vi "attempt path fix.vi"(9 "other possible paths":path[](array[path]), 10 "working directory":path, 11 "path to fix":path) -> (3 "path out":path)   [LabVIEW 2018]
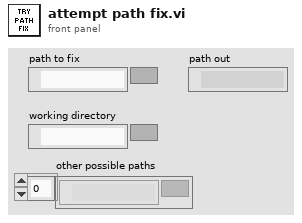
[diagram p1: front panel]
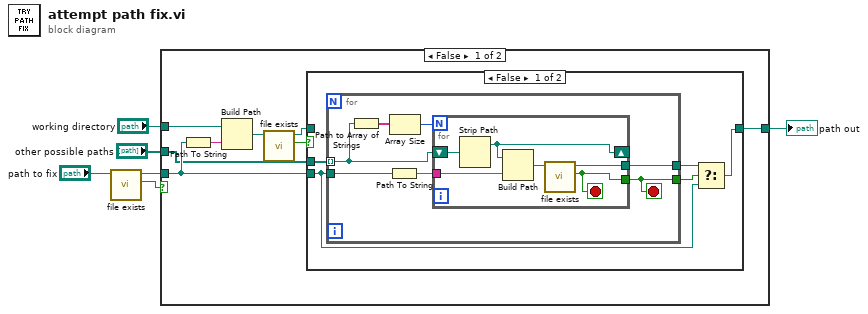
[diagram p0: block diagram]
diagram:
  n1 = call "file exists.vi"("Path in"="path to fix") -> ("file exists"=w5:bool, "Path out"=w3:path)  [unwired: 9 in]
  n2 = case shown="False" w5 {
    tunnel: [w9 w34] -> w4
    tunnel: w3 -> [w11 w34]
    tunnel: "working directory" -> [w13 _]
    tunnel: "other possible paths" -> [w8 _]
    frame False {
      n3 = Path To String(path=w11) -> (string=w14:string)
      n4 = Build Path(base path=w13, name or relative path=w14) -> (appended path=w12:path)
      n5 = call "file exists.vi"("Path in"=w12) -> ("file exists"=w10:bool, "Path out"=w7:path)  [unwired: 9 in]
      n6 = case shown="False" w10 {
        tunnel: w11 -> [w17 _]
        tunnel: [w15 w33] -> w9
        tunnel: w8 -> [w19 _]
        tunnel: w7 -> [_ w33]
        frame False {
          n7 = for {
            tunnel: w19 -> [w23] mode=indexing
            tunnel: [w20] -> w18
            tunnel: w17 -> [w22]
            tunnel: [w21] -> w16
            stop <- w20 stop-if-true
            n8 = Path to Array of Strings(0:w23) -> (2:w26:string[])  [unwired: 1 out]
            n9 = Path To String(path=w22) -> (string=w24:string)
            n10 = Array Size(array=w26) -> (size(s)=w25:i32)
            n11 = for {
              N: w25 -> [_]
              tunnel: w24 -> [w30]
              shift-right: [w31] -> _
              shift-left: w23 -> [w32]
              tunnel: [w28] -> w20
              tunnel: [w27] -> w21
              stop <- w28 stop-if-true
              n12 = Strip Path(path=w32) -> (stripped path=w31:path)  [unwired: 1 out]
              n13 = Build Path(base path=w31, name or relative path=w30) -> (appended path=w29:path)
              n14 = call "file exists.vi"("Path in"=w29) -> ("file exists"=w28:bool, "Path out"=w27:path)  [unwired: 9 in]
            }
          }
          n15 = Select(t=w16, s=w18, f=w17) -> (s? t:f=w15:path)
        }
        frame True {
        }
      }
    }
    frame True {
    }
  }
  "path out" <- w4
